vi "NXT M string.vi"(0 "string":string, 1 "error in":errorcluster) -> (2 "Motor":u16, 3 "Rudder":u16, 4 "error out":errorcluster)   [LabVIEW 2012, in "ENGR3390 Tug Boat.lvrbt"]
doc: "This VI parses the values of a string passed as a \"M\" from the PC. It is meant for manual control."
uses:
  ENGR3390 Tug Boat.lvrbt
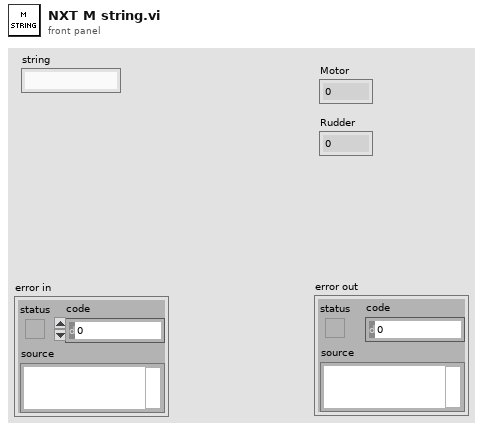
[diagram p1: front panel]
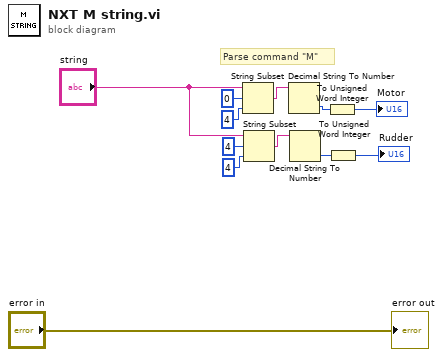
[diagram p0: block diagram]
diagram:
  # "Parse command \"M\""
  n1 = String Subset(string="string", offset (0)=0, length (rest)=4 ("length (rest)")) -> (substring=w12:string)
  n2 = String Subset(string="string", offset (0)=4, length (rest)=4 ("length (rest)")) -> (substring=w6:string)
  n3 = Decimal String To Number(string=w12) -> (number=w9:i32)  [unwired: 2 in, 1 out]
  n4 = Decimal String To Number(string=w6) -> (number=w5:i32)  [unwired: 2 in, 1 out]
  n5 = To Unsigned Word Integer(number=w9) -> (unsigned 16bit integer=→"Motor":u16)
  n6 = To Unsigned Word Integer(number=w5) -> (unsigned 16bit integer=→"Rudder":u16)
  "error out" <- "error in"
